vi "GetData.vi"(8 "file (use dialog) 2":path, 11 "file (use dialog)":path) -> (1 "Path Playback/Direction":T2, 2 "Trajectory Limits":T1, 3 "Trajectory Data":T5(array[cluster]), 4 "Commands":cluster{"Time (s)":dbl, T3, bool}[](array[cluster]), 5 "Points":cluster{"x":dbl, "y":dbl, "th":dbl}[](array[cluster]), 6 "Description":string, 7 "Path Time and Distance":cluster{"Time (s)":dbl, "Distance (ft)":dbl})   [LabVIEW 2019]
doc: "Getting trajectory data from the roboRio"
uses:
  Pathinator/bordeaux-pathinator/Bordeaux/Command Stuff/Single Cmd Info.ctl
  <vilib>/picture/picture.llb/imagedata.ctl
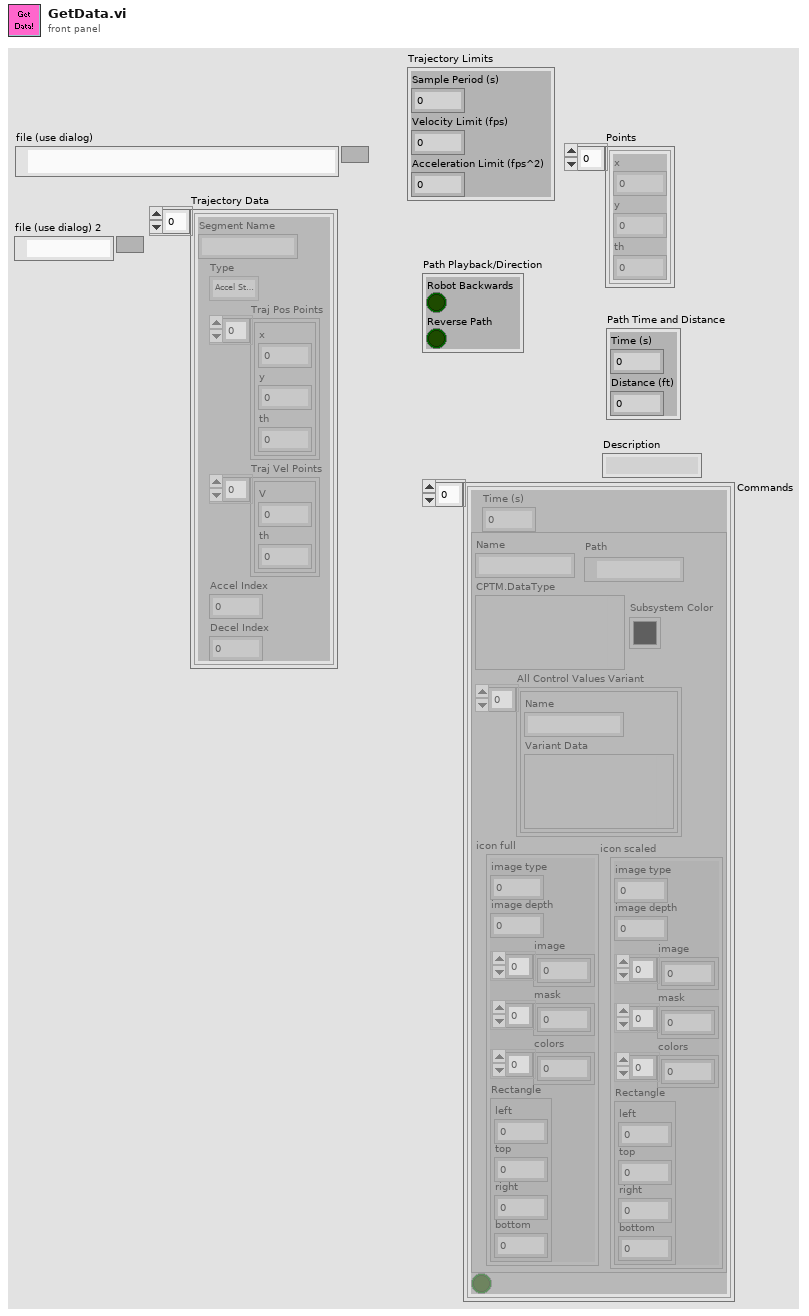
[diagram p1: front panel]
types:
  T1 = cluster{"Sample Period (s)":dbl, "Velocity Limit (fps)":dbl, "Acceleration Limit (fps^2)":dbl}
  T2 = cluster{"Robot Backwards":bool, "Reverse Path":bool}
  T3 = typedef "Single Cmd Info.ctl" = cluster{"Name":string, "CPTM.DataType":variant, "All Control Values Variant":cluster{"Name":string, "Variant Data":variant}[], "icon full":T4, "icon scaled":T4, "Path":path, "Subsystem Color":u32}
  T4 = typedef "imagedata.ctl" = cluster{"image type":i32, "image depth":i32, "image":u8[], "mask":u8[], "colors":u32[], "Rectangle":cluster{"left":i16, "top":i16, "right":i16, "bottom":i16}}
  T5 = cluster{"Segment Name":string, "Type":enum16{"Accel Straight", "Const Straight", "Blend", "Circle"}, "Traj Pos Points":cluster{"x":dbl, "y":dbl, "th":dbl}[], "Traj Vel Points":cluster{"V":dbl, "th":dbl}[], "Accel Index":i32, "Decel Index":i32}[]
  T6 = cluster{"Sample Period (s)":dbl, "Limits":cluster{"Velocity (fps)":dbl, "Acceleration (fps^2)":dbl, "Jerk (fps^3)":dbl}, "Conditions":cluster{"vInitial (fps)":dbl, "vFinal (fps)":dbl}}
  T7 = cluster{"Velocity Limit (fps)":dbl, "Sample Period (s)":dbl, "Acceleration Limit (fps^2)":dbl}
  T8 = cluster{"Sample Period (s)":dbl, "Limits":cluster{"Velocity (fps)":dbl, "Acceleration (fps^2)":dbl, "Jerk (fps^3)":dbl}, "Conditions":cluster{"vInitial (fps)":dbl, "vFinal (fps)":dbl}, "Min Rads":dbl[]}
  T9 = cluster{"Sample Period (s)":dbl, "Limits":cluster{"Velocity (fps)":dbl, "Acceleration (fps^2)":dbl, "Jerk (fps^3)":dbl}, "Conditions":cluster{"vInitial (fps)":dbl, "vFinal (fps)":dbl}, "Angular Accelerations":cluster{"Angular \nAccelerations":dbl[], "Override Limits?":bool[]}}
  T10 = cluster{"Time into Path":dbl, "System":u16, "Item Selected?":bool, "System Selection":u16}[]
  T11 = cluster{"Velocity (fps)":dbl, "Acceleration (fps^2)":dbl, "Jerk (fps^3)":dbl}
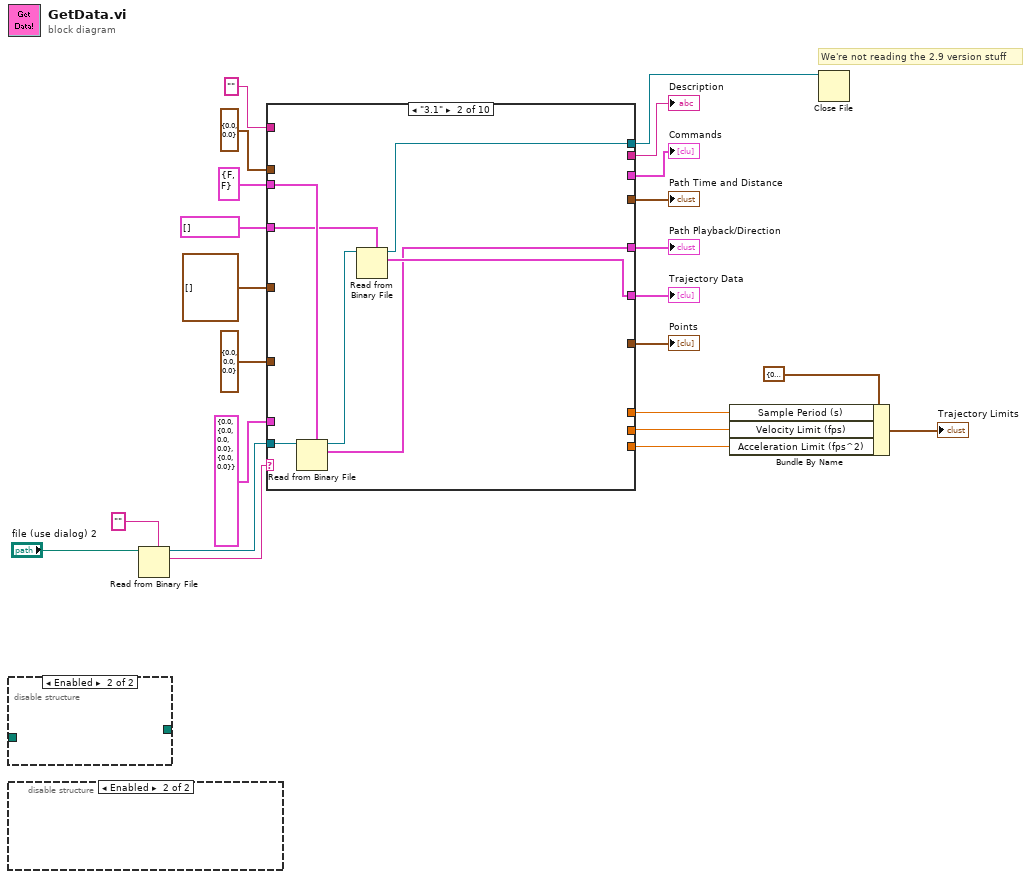
[diagram p0: block diagram]
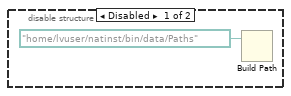
[diagram p2: hidden frame]
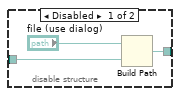
[diagram p3: hidden frame]
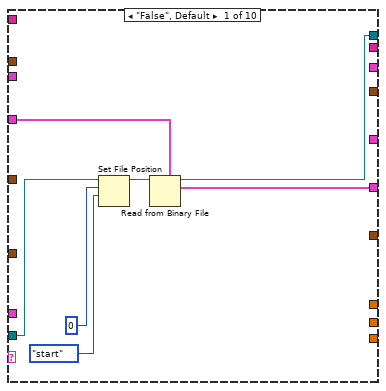
[diagram p4: hidden frame]
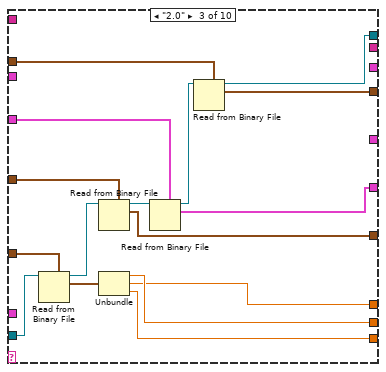
[diagram p5: hidden frame]
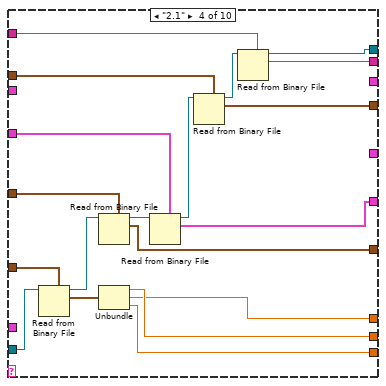
[diagram p6: hidden frame]
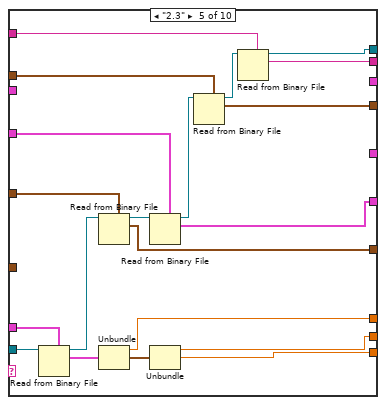
[diagram p7: hidden frame]
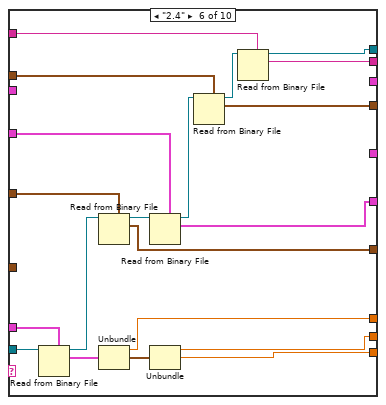
[diagram p8: hidden frame]
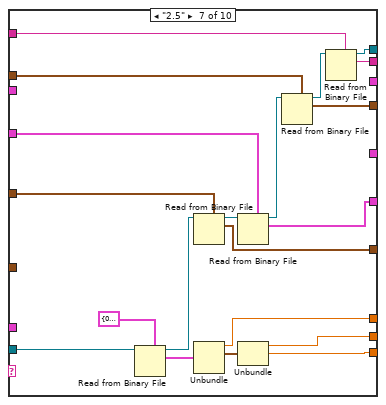
[diagram p9: hidden frame]
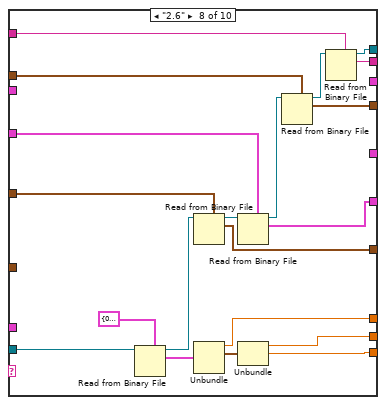
[diagram p10: hidden frame]
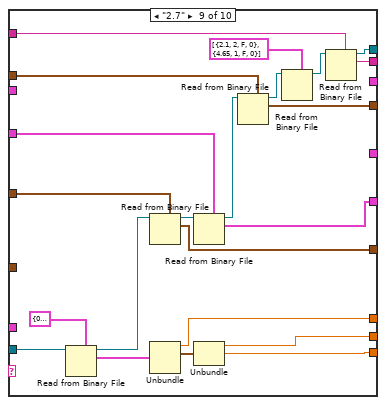
[diagram p11: hidden frame]
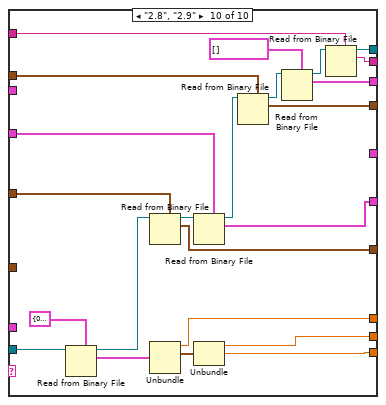
[diagram p12: hidden frame]
diagram:
  # "We're not reading the 2.9 version stuff"
  n1 = disable-structure shown="Enabled" {
    disable-tunnel: [w25 _] -> _
    disable-tunnel: _ -> [w24 _]
    frame Disabled {
      n2 = Build Path(base path="file (use dialog)", name or relative path=w24) -> (appended path=w25:path)
    }
    frame Enabled {
    }
  }
  n3 = disable-structure shown="Enabled" {
    frame Disabled {
      n4 = Build Path(base path=path "/home/lvuser/natinst/bin/data/Paths") -> (name or relative path=w27:string)  [unwired: 1 out]
    }
    frame Enabled {
    }
  }
  n5 = Read from Binary File(5:"", 11:"file (use dialog) 2") -> (2:w22:string, 3:w21:refnum<file>)  [unwired: 4 in, 2 out]
  n6 = case shown="\"3.1\"" w22 {
    tunnel: w21 -> [w30 w38 w57 w76 w96 w116 w136 w156 w178 w201]
    tunnel: T7 {"Velocity Limit (fps)"=0.0, "Sample Period (s)"=0.0, "Acceleration Limit (fps^2)"=0.0} -> [_ _ w56 w75 _ _ _ _ _ _]
    tunnel: cluster{"x":dbl, "y":dbl, "th":dbl}[] [] ("Points") -> [_ _ w54 w73 w94 w114 w134 w154 w176 w199]
    tunnel: [_ _ w53 w72 w93 w113 w133 w153 w175 w198] -> w15
    tunnel: T5 [] ("Trajectory Data") -> [w32 w41 w52 w71 w92 w112 w132 w152 w174 w197]
    tunnel: [w31 w40 w50 w69 w90 w110 w130 w150 w172 w195] -> w14
    tunnel: cluster{"Time (s)":dbl, "Distance (ft)":dbl} {"Time (s)"=0.0, "Distance (ft)"=0.0} -> [_ _ w49 w68 w89 w109 w129 w149 w171 w194]
    tunnel: [_ _ w47 w66 w87 w107 w127 w147 w169 w192] -> w13
    tunnel: [w29 w36 w46 w61 w85 w105 w125 w145 w168 w191] -> w19
    tunnel: [_ _ w45 w65 w80 w100 w121 w141 w164 w187] -> w3
    tunnel: [_ _ w44 w64 w78 w98 w119 w139 w162 w185] -> w4
    tunnel: [_ _ w43 w63 w79 w99 w120 w140 w163 w186] -> w2
    tunnel: "" -> [_ _ _ w60 w84 w104 w124 w144 w167 w190]
    tunnel: [_ _ _ w59 w83 w103 w123 w143 w166 w189] -> w11
    tunnel: T6 {"Sample Period (s)"=0.0, "Limits"={"Velocity (fps)"=0.0, "Acceleration (fps^2)"=0.0, "Jerk (fps^3)"=0.0}, "Conditions"={"vInitial (fps)"=0.0, "vFinal (fps)"=0.0}} -> [_ _ _ _ w82 w102 _ _ _ _]
    tunnel: [_ _ _ _ _ _ _ _ _ w180] -> w9
    tunnel: T2 {"Robot Backwards"=FALSE, "Reverse Path"=FALSE} ("Cluster") -> [_ w42 _ _ _ _ _ _ _ _]
    tunnel: [_ w39 _ _ _ _ _ _ _ _] -> w6
    frame "False", Default {
      n7 = Set File Position(offset (in bytes) (0)=i64 0, refnum=w30, from (0:start)=enum16{"start", "end", "current"}."start") -> (refnum out=w33:refnum<file>)  [unwired: 1 in, 1 out]
      n8 = Read from Binary File(5:w32, 11:w33) -> (2:w31:T5, 3:w29:refnum<file>)  [unwired: 4 in, 2 out]
    }
    frame "3.1" {
      n9 = Read from Binary File(5:w42, 11:w38) -> (2:w39:T2, 3:w37:refnum<file>)  [unwired: 4 in, 2 out]
      n10 = Read from Binary File(5:w41, 11:w37) -> (2:w40:T5, 3:w36:refnum<file>)  [unwired: 4 in, 2 out]
    }
    frame "2.0" {
      n11 = Read from Binary File(5:w56, 11:w57) -> (2:w58:T7, 3:w55:refnum<file>)  [unwired: 4 in, 2 out]
      n12 = Read from Binary File(5:w54, 11:w55) -> (2:w53:cluster{"x":dbl, "y":dbl, "th":dbl}[], 3:w51:refnum<file>)  [unwired: 4 in, 2 out]
      n13 = Unbundle(w58) -> ("Velocity Limit (fps)"=w45:dbl, "Sample Period (s)"=w44:dbl, "Acceleration Limit (fps^2)"=w43:dbl)
      n14 = Read from Binary File(5:w52, 11:w51) -> (2:w50:T5, 3:w48:refnum<file>)  [unwired: 4 in, 2 out]
      n15 = Read from Binary File(5:w49, 11:w48) -> (2:w47:cluster{"Time (s)":dbl, "Distance (ft)":dbl}, 3:w46:refnum<file>)  [unwired: 4 in, 2 out]
    }
    frame "2.1" {
      n16 = Read from Binary File(5:w75, 11:w76) -> (2:w77:T7, 3:w74:refnum<file>)  [unwired: 4 in, 2 out]
      n17 = Read from Binary File(5:w73, 11:w74) -> (2:w72:cluster{"x":dbl, "y":dbl, "th":dbl}[], 3:w70:refnum<file>)  [unwired: 4 in, 2 out]
      n18 = Unbundle(w77) -> ("Velocity Limit (fps)"=w65:dbl, "Sample Period (s)"=w64:dbl, "Acceleration Limit (fps^2)"=w63:dbl)
      n19 = Read from Binary File(5:w71, 11:w70) -> (2:w69:T5, 3:w67:refnum<file>)  [unwired: 4 in, 2 out]
      n20 = Read from Binary File(5:w68, 11:w67) -> (2:w66:cluster{"Time (s)":dbl, "Distance (ft)":dbl}, 3:w62:refnum<file>)  [unwired: 4 in, 2 out]
      n21 = Read from Binary File(5:w60, 11:w62) -> (2:w59:string, 3:w61:refnum<file>)  [unwired: 4 in, 2 out]
    }
    frame "2.3" {
      n22 = Read from Binary File(5:w82, 11:w96) -> (2:w97:T6, 3:w95:refnum<file>)  [unwired: 4 in, 2 out]
      n23 = Read from Binary File(5:w94, 11:w95) -> (2:w93:cluster{"x":dbl, "y":dbl, "th":dbl}[], 3:w91:refnum<file>)  [unwired: 4 in, 2 out]
      n24 = Unbundle(w97) -> ("Sample Period (s)"=w78:dbl, "Limits"=w81:T11)  [unwired: 1 out]
      n25 = Read from Binary File(5:w92, 11:w91) -> (2:w90:T5, 3:w88:refnum<file>)  [unwired: 4 in, 2 out]
      n26 = Unbundle(w81) -> ("Velocity (fps)"=w80:dbl, "Acceleration (fps^2)"=w79:dbl)  [unwired: 1 out]
      n27 = Read from Binary File(5:w89, 11:w88) -> (2:w87:cluster{"Time (s)":dbl, "Distance (ft)":dbl}, 3:w86:refnum<file>)  [unwired: 4 in, 2 out]
      n28 = Read from Binary File(5:w84, 11:w86) -> (2:w83:string, 3:w85:refnum<file>)  [unwired: 4 in, 2 out]
    }
    frame "2.4" {
      n29 = Read from Binary File(5:w102, 11:w116) -> (2:w117:T6, 3:w115:refnum<file>)  [unwired: 4 in, 2 out]
      n30 = Read from Binary File(5:w114, 11:w115) -> (2:w113:cluster{"x":dbl, "y":dbl, "th":dbl}[], 3:w111:refnum<file>)  [unwired: 4 in, 2 out]
      n31 = Unbundle(w117) -> ("Sample Period (s)"=w98:dbl, "Limits"=w101:T11)  [unwired: 1 out]
      n32 = Read from Binary File(5:w112, 11:w111) -> (2:w110:T5, 3:w108:refnum<file>)  [unwired: 4 in, 2 out]
      n33 = Unbundle(w101) -> ("Velocity (fps)"=w100:dbl, "Acceleration (fps^2)"=w99:dbl)  [unwired: 1 out]
      n34 = Read from Binary File(5:w109, 11:w108) -> (2:w107:cluster{"Time (s)":dbl, "Distance (ft)":dbl}, 3:w106:refnum<file>)  [unwired: 4 in, 2 out]
      n35 = Read from Binary File(5:w104, 11:w106) -> (2:w103:string, 3:w105:refnum<file>)  [unwired: 4 in, 2 out]
    }
    frame "2.5" {
      n36 = Read from Binary File(5:T8 {"Sample Period (s)"=0.0, "Limits"={"Velocity (fps)"=0.0, "Acceleration (fps^2)"=0.0, "Jerk (fps^3)"=0.0}, "Conditions"={"vInitial (fps)"=0.0, "vFinal (fps)"=0.0}, "Min Rads"=[20.0, 20.0, 20.0, 20.0, 20.0]}, 11:w136) -> (2:w137:T8, 3:w135:refnum<file>)  [unwired: 4 in, 2 out]
      n37 = Read from Binary File(5:w134, 11:w135) -> (2:w133:cluster{"x":dbl, "y":dbl, "th":dbl}[], 3:w131:refnum<file>)  [unwired: 4 in, 2 out]
      n38 = Unbundle(w137) -> ("Sample Period (s)"=w119:dbl, "Limits"=w122:T11)  [unwired: 2 out]
      n39 = Read from Binary File(5:w132, 11:w131) -> (2:w130:T5, 3:w128:refnum<file>)  [unwired: 4 in, 2 out]
      n40 = Unbundle(w122) -> ("Velocity (fps)"=w121:dbl, "Acceleration (fps^2)"=w120:dbl)  [unwired: 1 out]
      n41 = Read from Binary File(5:w129, 11:w128) -> (2:w127:cluster{"Time (s)":dbl, "Distance (ft)":dbl}, 3:w126:refnum<file>)  [unwired: 4 in, 2 out]
      n42 = Read from Binary File(5:w124, 11:w126) -> (2:w123:string, 3:w125:refnum<file>)  [unwired: 4 in, 2 out]
    }
    frame "2.6" {
      n43 = Read from Binary File(5:T9 {"Sample Period (s)"=0.0, "Limits"={"Velocity (fps)"=0.0, "Acceleration (fps^2)"=0.0, "Jerk (fps^3)"=0.0}, "Conditions"={"vInitial (fps)"=0.0, "vFinal (fps)"=0.0}, "Angular Accelerations"={"Angular \nAccelerations"=[], "Override Limits?"=[]}}, 11:w156) -> (2:w157:T9, 3:w155:refnum<file>)  [unwired: 4 in, 2 out]
      n44 = Read from Binary File(5:w154, 11:w155) -> (2:w153:cluster{"x":dbl, "y":dbl, "th":dbl}[], 3:w151:refnum<file>)  [unwired: 4 in, 2 out]
      n45 = Unbundle(w157) -> ("Sample Period (s)"=w139:dbl, "Limits"=w142:T11)  [unwired: 2 out]
      n46 = Read from Binary File(5:w152, 11:w151) -> (2:w150:T5, 3:w148:refnum<file>)  [unwired: 4 in, 2 out]
      n47 = Unbundle(w142) -> ("Velocity (fps)"=w141:dbl, "Acceleration (fps^2)"=w140:dbl)  [unwired: 1 out]
      n48 = Read from Binary File(5:w149, 11:w148) -> (2:w147:cluster{"Time (s)":dbl, "Distance (ft)":dbl}, 3:w146:refnum<file>)  [unwired: 4 in, 2 out]
      n49 = Read from Binary File(5:w144, 11:w146) -> (2:w143:string, 3:w145:refnum<file>)  [unwired: 4 in, 2 out]
    }
    frame "2.7" {
      n50 = Read from Binary File(5:T9 {"Sample Period (s)"=0.0, "Limits"={"Velocity (fps)"=0.0, "Acceleration (fps^2)"=0.0, "Jerk (fps^3)"=0.0}, "Conditions"={"vInitial (fps)"=0.0, "vFinal (fps)"=0.0}, "Angular Accelerations"={"Angular \nAccelerations"=[], "Override Limits?"=[]}}, 11:w178) -> (2:w179:T9, 3:w177:refnum<file>)  [unwired: 4 in, 2 out]
      n51 = Read from Binary File(5:w176, 11:w177) -> (2:w175:cluster{"x":dbl, "y":dbl, "th":dbl}[], 3:w173:refnum<file>)  [unwired: 4 in, 2 out]
      n52 = Unbundle(w179) -> ("Sample Period (s)"=w162:dbl, "Limits"=w165:T11)  [unwired: 2 out]
      n53 = Read from Binary File(5:w174, 11:w173) -> (2:w172:T5, 3:w170:refnum<file>)  [unwired: 4 in, 2 out]
      n54 = Unbundle(w165) -> ("Velocity (fps)"=w164:dbl, "Acceleration (fps^2)"=w163:dbl)  [unwired: 1 out]
      n55 = Read from Binary File(5:w171, 11:w170) -> (2:w169:cluster{"Time (s)":dbl, "Distance (ft)":dbl}, 3:w160:refnum<file>)  [unwired: 4 in, 2 out]
      n56 = Read from Binary File(5:T10 [{"Time into Path"=2.1, "System"=2, "Item Selected?"=FALSE, "System Selection"=0}, {"Time into Path"=4.65, "System"=1, "Item Selected?"=FALSE, "System Selection"=0}] ("Commands"), 11:w160) -> (3:w159:refnum<file>)  [unwired: 4 in, 3 out]
      n57 = Read from Binary File(5:w167, 11:w159) -> (2:w166:string, 3:w168:refnum<file>)  [unwired: 4 in, 2 out]
    }
    frame "2.8", "2.9" {
      n58 = Read from Binary File(5:T9 {"Sample Period (s)"=0.0, "Limits"={"Velocity (fps)"=0.0, "Acceleration (fps^2)"=0.0, "Jerk (fps^3)"=0.0}, "Conditions"={"vInitial (fps)"=0.0, "vFinal (fps)"=0.0}, "Angular Accelerations"={"Angular \nAccelerations"=[], "Override Limits?"=[]}}, 11:w201) -> (2:w202:T9, 3:w200:refnum<file>)  [unwired: 4 in, 2 out]
      n59 = Read from Binary File(5:w199, 11:w200) -> (2:w198:cluster{"x":dbl, "y":dbl, "th":dbl}[], 3:w196:refnum<file>)  [unwired: 4 in, 2 out]
      n60 = Unbundle(w202) -> ("Sample Period (s)"=w185:dbl, "Limits"=w188:T11)  [unwired: 2 out]
      n61 = Read from Binary File(5:w197, 11:w196) -> (2:w195:T5, 3:w193:refnum<file>)  [unwired: 4 in, 2 out]
      n62 = Unbundle(w188) -> ("Velocity (fps)"=w187:dbl, "Acceleration (fps^2)"=w186:dbl)  [unwired: 1 out]
      n63 = Read from Binary File(5:w194, 11:w193) -> (2:w192:cluster{"Time (s)":dbl, "Distance (ft)":dbl}, 3:w183:refnum<file>)  [unwired: 4 in, 2 out]
      n64 = Read from Binary File(5:cluster{"Time (s)":dbl, T3, bool}[] [], 11:w183) -> (2:w180:cluster{"Time (s)":dbl, T3, bool}[], 3:w182:refnum<file>)  [unwired: 4 in, 2 out]
      n65 = Read from Binary File(5:w190, 11:w182) -> (2:w189:string, 3:w191:refnum<file>)  [unwired: 4 in, 2 out]
    }
  }
  "Points" <- w15
  "Trajectory Data" <- w14
  "Path Time and Distance" <- w13
  "Description" <- w11
  "Commands" <- w9
  "Path Playback/Direction" <- w6
  n66 = Bundle By Name(cluster=T1 {"Sample Period (s)"=0.0, "Velocity Limit (fps)"=0.0, "Acceleration Limit (fps^2)"=0.0} ("input cluster"), "Sample Period (s)"=w4, "Velocity Limit (fps)"=w3, "Acceleration Limit (fps^2)"=w2) -> (→"Trajectory Limits":T1)
  n67 = Close File(refnum=w19) -> ()  [unwired: 1 in, 2 out]
